vi "KProp-Table to Cluster.vi"(0 "Anything":variant, 7 "Rows":T1[](array[typedef]), 11 "Error In":errorcluster) -> (4 "variant":variant, 15 "Error Out":errorcluster)   [LabVIEW 2020, in "KPropertyTable.xctl"]
uses:
  KPropertyTable.xctl
  RowData.ctl
  DataType.ctl
  <vilib>/Utility/Data Type/NI_Data Type.lvlib
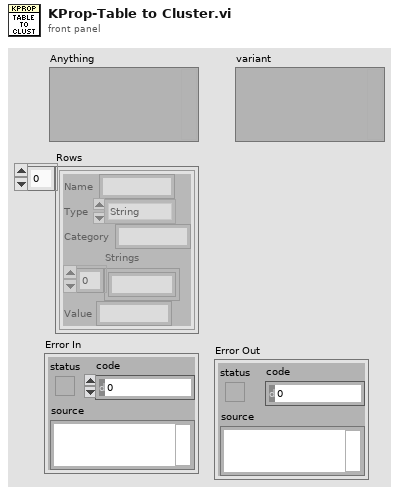
[diagram p1: front panel]
types:
  T1 = typedef "KPropertyTable.xctl/RowData.ctl" = cluster{"Name":string, "Type":T2, "Category":string, "Strings":string[], "Value":string}
  T2 = typedef "KPropertyTable.xctl/DataType.ctl" = enum16{"String", "Enum", "Int", "Double", "Boolean", "Ring", "Formula"}
  T3 = typedef "NI_Data Type.lvlib/Data Type.ctl" = enum8{"Invalid Type", "Void", "I8", "I16", "I32", "I64", "U8", "U16", "U32", "U64", "Single Float", "Double Float", "Extended Float", "Single Complex", "Double Complex", "Extended Complex", "Enum U8", "Enum U16", "Enum U32", "Enum U64", "Single Float With Unit", "Double Float With Unit", "Extended Float With Unit", "Single Complex with Unit", "Double Complex with Unit", "Extended Complex with Unit", "Boolean", "String", "Path", "Picture", "Tag", "Array", "Cluster", "Variant", "LV Variant", "Waveform", "Timestamp", "Digital Waveform", "Digital Data", "ExpressData", "Refnum", "External Data", "VI", "Poly VI", "LabVIEW Class Instance", "Fixed Point", "Set Collection", "Map Collection"}
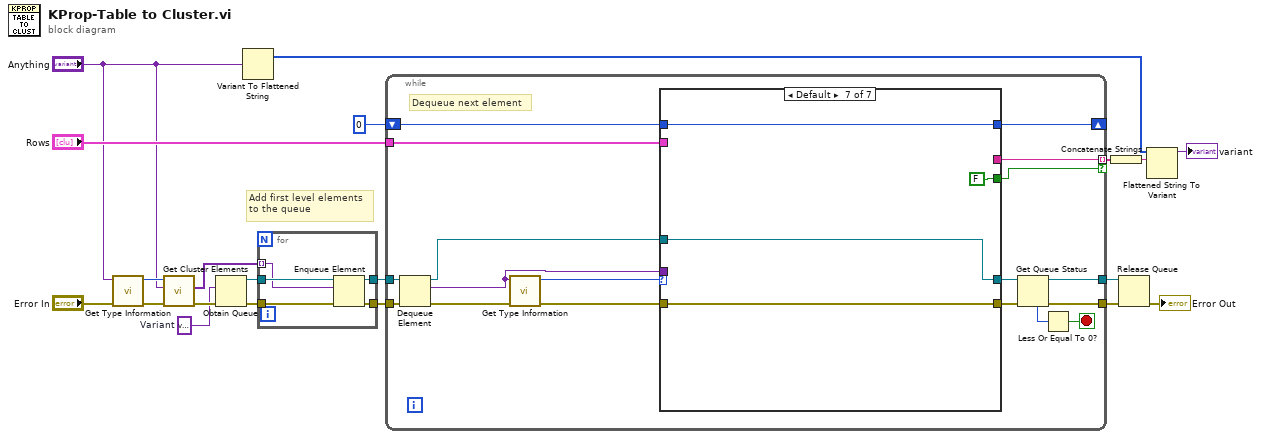
[diagram p0: block diagram]
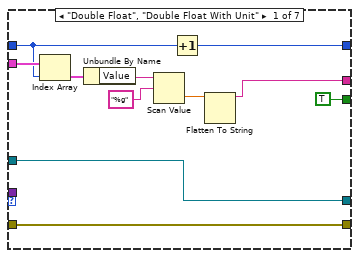
[diagram p2: hidden frame]
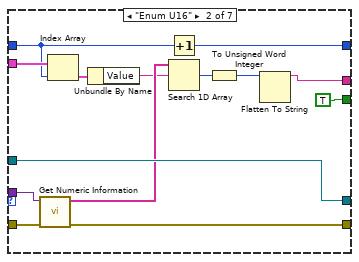
[diagram p3: hidden frame]
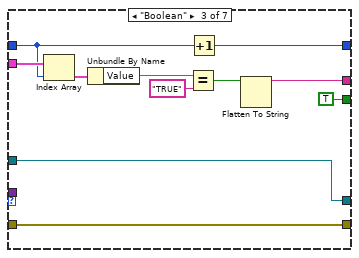
[diagram p4: hidden frame]
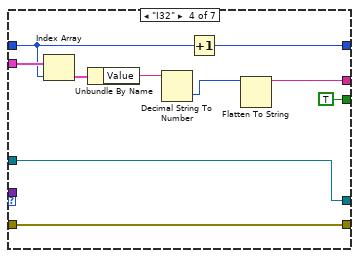
[diagram p5: hidden frame]
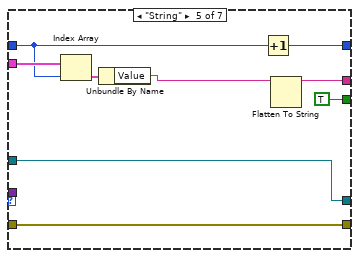
[diagram p6: hidden frame]
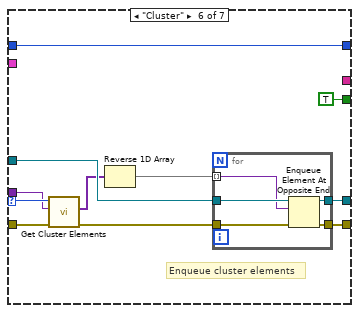
[diagram p7: hidden frame]
diagram:
  w1 = variant  # Variant
  # "Add first level elements\nto the queue"
  n1 = call <vilib>:"Get Type Information.vi"("error in (no error)"="Error In", "variant"="Anything") -> ("error out"=w16:errorcluster, "type"=w20:T3)  [unwired: 5 in, 3 out]
  n2 = call "Get Cluster Elements.vi"("Error In"=w16, "Cluster"="Anything", "Type Enum (Cluster)"=w20) -> ("Error Out"=w18:errorcluster, "Cluster Elements"=w17:variant[])  [unwired: 7 in]
  n3 = Obtain Queue(element data type=w1, error in (no error)=w18) -> (queue out=w9:refnum<queue>, error out=w10:errorcluster)  [unwired: 3 in, 1 out]
  n4 = Variant To Flattened String(Variant="Anything") -> (1:w4:i16[])  [unwired: 1 out]
  n5 = for {
    tunnel: w9 -> [w25]
    tunnel: w10 -> [w24]
    tunnel: [w23] -> w11
    tunnel: [w22] -> w12
    tunnel: w17 -> [w21] mode=indexing
    n6 = Enqueue Element(queue=w25, element=w21, error in (no error)=w24) -> (queue out=w22:refnum<queue>, error out=w23:errorcluster)  [unwired: 1 in, 1 out]
  }
  n7 = while {
    tunnel: w11 -> [w43]
    tunnel: [w40] -> w13
    tunnel: w12 -> [w41]
    tunnel: [w37] -> w14
    tunnel: "Rows" -> [w31]
    shift-right: [w29] -> _
    shift-left: 0 -> [w30]
    tunnel: [w28] -> w5 mode=indexing if=w27
    stop <- w38 stop-if-true
    # "Dequeue next element"
    n8 = Dequeue Element(queue=w41, error in (no error)=w43) -> (queue out=w34:refnum<queue>, element=w26:variant, error out=w42:errorcluster)  [unwired: 1 in, 1 out]
    n9 = call <vilib>:"Get Type Information.vi"("error in (no error)"=w42, "variant"=w26) -> ("error out"=w32:errorcluster, "type"=w36:T3)  [unwired: 5 in, 3 out]
    n10 = case shown="Default" w36 {
      selector: w36 -> [_ _ _ _ _ w103 _]
      tunnel: [w54 w68 w79 w89 w98 w107 w118] -> w35
      tunnel: w34 -> [w54 w68 w79 w89 w98 w108 w118]
      tunnel: [w53 w64 w69 w82 w97 w109 w117] -> w33
      tunnel: w32 -> [w53 w67 w69 w82 w97 w105 w117]
      tunnel: w26 -> [_ w66 _ _ _ w102 _]
      tunnel: [TRUE TRUE TRUE TRUE TRUE TRUE FALSE] -> w27
      tunnel: w31 -> [w51 w63 w77 w87 w95 _ _]
      tunnel: w30 -> [w50 w62 w76 w86 w94 w99 w115]
      tunnel: [w44 w61 w70 w83 w93 w99 w115] -> w29
      tunnel: [w45 w55 w71 w84 w92 _ _] -> w28
      frame "Double Float", "Double Float With Unit" {
        n11 = Index Array(array=w51, index=w50) -> (element=w49:T1)
        n12 = Unbundle By Name(w49) -> ("Value"=w48:string)
        n13 = Scan Value(string=w48, format string="%g") -> (value=w46:dbl)  [unwired: 1 in, 1 out]
        n14 = Increment(x=w50) -> (x+1=w44:i32)
        n15 = Flatten To String(anything=w46) -> (data string=w45:string)  [unwired: 3 in, 2 out]
      }
      frame "Enum U16" {
        n16 = call <vilib>:"Get Numeric Information.vi"("error in (no error)"=w67, "variant"=w66) -> ("error out"=w64:errorcluster, "enum names"=w59:string[])  [unwired: 6 in, 2 out]
        n17 = Index Array(array=w63, index=w62) -> (element=w60:T1)
        n18 = Unbundle By Name(w60) -> ("Value"=w58:string)
        n19 = Increment(x=w62) -> (x+1=w61:i32)
        n20 = Search 1D Array(1D array=w59, element=w58) -> (index of element=w57:i32)  [unwired: 1 in]
        n21 = To Unsigned Word Integer(number=w57) -> (unsigned 16bit integer=w56:u16)
        n22 = Flatten To String(anything=w56) -> (data string=w55:string)  [unwired: 3 in, 2 out]
      }
      frame "Boolean" {
        n23 = Index Array(array=w77, index=w76) -> (element=w75:T1)
        n24 = Unbundle By Name(w75) -> ("Value"=w73:string)
        n25 = Equal?(x=w73, y="TRUE") -> (x = y?=w72:bool)
        n26 = Increment(x=w76) -> (x+1=w70:i32)
        n27 = Flatten To String(anything=w72) -> (data string=w71:string)  [unwired: 3 in, 2 out]
      }
      frame "I32" {
        n28 = Index Array(array=w87, index=w86) -> (element=w85:T1)
        n29 = Unbundle By Name(w85) -> ("Value"=w81:string)
        n30 = Decimal String To Number(string=w81) -> (number=w80:i32)  [unwired: 2 in, 1 out]
        n31 = Increment(x=w86) -> (x+1=w83:i32)
        n32 = Flatten To String(anything=w80) -> (data string=w84:string)  [unwired: 3 in, 2 out]
      }
      frame "String" {
        n33 = Index Array(array=w95, index=w94) -> (element=w91:T1)
        n34 = Unbundle By Name(w91) -> ("Value"=w90:string)
        n35 = Increment(x=w94) -> (x+1=w93:i32)
        n36 = Flatten To String(anything=w90) -> (data string=w92:string)  [unwired: 3 in, 2 out]
      }
      frame "Cluster" {
        # "Enqueue cluster elements"
        n37 = call "Get Cluster Elements.vi"("Error In"=w105, "Cluster"=w102, "Type Enum (Cluster)"=w103) -> ("Error Out"=w104:errorcluster, "Cluster Elements"=w101:variant[])  [unwired: 7 in]
        n38 = Reverse 1D Array(array=w101) -> (reversed array=w106:variant[])
        n39 = for {
          tunnel: w108 -> [w114]
          tunnel: w104 -> [w113]
          tunnel: [w112] -> w109
          tunnel: [w111] -> w107
          tunnel: w106 -> [w110] mode=indexing
          n40 = Enqueue Element At Opposite End(queue=w114, element=w110, error in (no error)=w113) -> (queue out=w111:refnum<queue>, error out=w112:errorcluster)  [unwired: 1 in, 1 out]
        }
      }
      frame Default {
      }
    }
    n41 = Get Queue Status(queue=w35, error in (no error)=w33) -> (queue out=w37:refnum<queue>, error out=w40:errorcluster, # elements in queue=w39:i32)  [unwired: 1 in, 5 out]
    n42 = Less Or Equal To 0?(x=w39) -> (x <= 0?=w38:bool)
  }
  n43 = Concatenate Strings(w5) -> (w2:string)
  n44 = Release Queue(queue=w14, error in (no error)=w13) -> (error out=→"Error Out":errorcluster)  [unwired: 1 in, 2 out]
  n45 = Flattened String To Variant(6:w2, 7:w4) -> (3:→"variant":variant)  [unwired: 1 in, 1 out]
